vi "Target.vi"() -> ()   [LabVIEW 2025]
uses:
  <vilib>/Platform/TimedLoop/XDataNode/timing_clust.ctl
  <vilib>/Platform/TimedLoop/XDataNode/nitl_modes.ctl
  <vilib>/Platform/TimedLoop/XDataNode/wakeup.ctl
  <vilib>/rvi/Emulation/niFpgaSctlEmulationGetInTimedLoop.vi
  <vilib>/rvi/Emulation/niFpgaEmulationReportErrorSimple.vi
  <vilib>/rvi/Emulation/niFpgaGetClockAttributes.vi
  <vilib>/rvi/Emulation/niFpgaCriticalErrorInLSC.vi
  <vilib>/rvi/linearAlgebra/MatrixMultiply/simVIs/SubVI/nifxpla_MatrixMultiply_SimMatrixSizes.vi
  <vilib>/rvi/linearAlgebra/MatrixMultiply/simVIs/SubVI/nifxpla_MatrixMultiply_Sim4WireAdapterVector.vi
  <vilib>/rvi/linearAlgebra/MatrixMultiply/simVIs/SubVI/nifxpla_MatrixMultiply_SimFrameHandShake.vi
  <vilib>/rvi/linearAlgebra/MatrixMultiply/simVIs/SubVI/nifxpla_MatrixMultiply_SimEndlessCounter.vi
  <vilib>/rvi/linearAlgebra/MatrixMultiply/simVIs/SubVI/nifxpla_MatrixMultiply_SimVectorDataBuffer.vi
  <vilib>/rvi/ClientSDK/Core/DevComputerLib/Private/Multiply(dfxp64).vi
  <vilib>/rvi/ClientSDK/Core/DevComputerLib/Private/Dfxp128ToDfxp256.vi
  <vilib>/rvi/ClientSDK/Core/DevComputerLib/Private/Add(dfxp256).vi
  <vilib>/rvi/ClientSDK/Core/DevComputerLib/Private/Subtract(dfxp256).vi
  <vilib>/rvi/ClientSDK/Core/DevComputerLib/Private/ToDfxp64(dfxp256).vi
  <vilib>/platform/TimedLoop/XDataNode/XDataNode.xnode
  <vilib>/rvi/linearAlgebra/MatrixMultiply/XNode/nifxpla_MatrixMultiply.xnode
  <vilib>/rvi/linearAlgebra/MatrixMultiply/simVIs/nifxpla_MatrixMultiply_SimTemplateEinEout.vi
  <vilib>/rvi/linearAlgebra/MatrixMultiply/simVIs/nifxpla_MatrixMultiply_SimTemplateEinVout.vi
  <vilib>/rvi/linearAlgebra/MatrixMultiply/simVIs/nifxpla_MatrixMultiply_SimTemplateVinEout.vi
  <vilib>/rvi/linearAlgebra/MatrixMultiply/simVIs/nifxpla_MatrixMultiply_SimTemplateVinVout.vi
  <vilib>/Platform/TimedLoop/XDataNode/XDNodeRunTimeDep.lvlib
panel:
  out "C1+B":fxp<+/-,33,17>[](array[numeric])
  out "C1":fxp<+/-,32,16>[](array[numeric])
  out "Cycle Count":i32
  out "C2+B":fxp<+/-,33,17>[](array[numeric])
  out "C2":fxp<+/-,32,16>[](array[numeric])
  out "Cycle Count 2":i32
  out "C3+B":fxp<+/-,33,17>[](array[numeric])
  out "C3":fxp<+/-,32,16>[](array[numeric])
  out "Cycle Count 3":i32
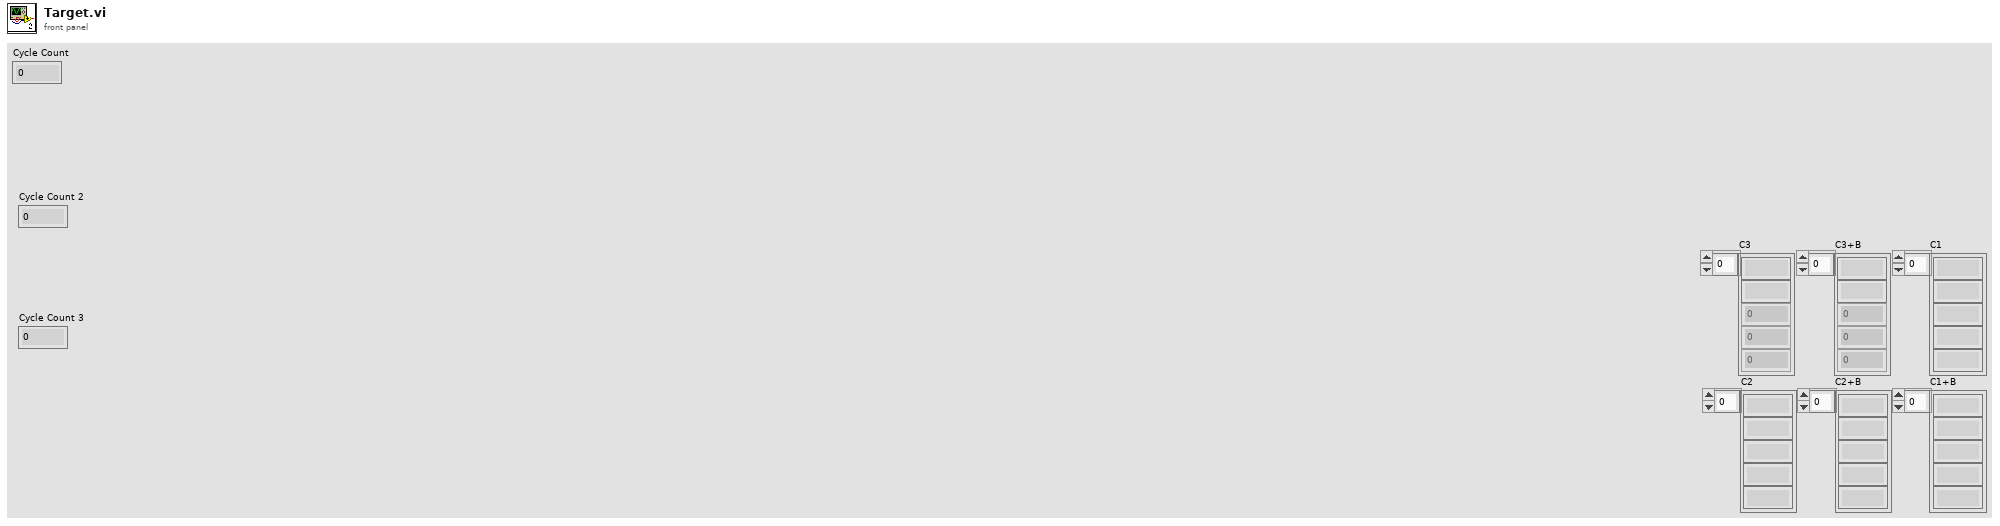
[diagram p1: front panel]
types:
  T1 = typedef "XDNodeRunTimeDep.lvlib/timing_clust.ctl" = cluster{"Expected End [f-1]":u64, "Actual End [f-1]":u64, "Finished Late? [f-1]":bool, "Expected End [i-1]":u64, "Actual End [i-1]":u64, "Finished Late? [i-1]":bool, "Expected Start [i]":u64, "Actual Start [i]":u64, "Expected Start [f]":u64, "Actual Start [f]":u64, "Source Name":string, "Structure Name":string, "Period":i64, "Deadline":i64, "Offset":i64, "Start":i64, "Priority":i32, "Timeout":i32, "Mode":T2, "Wakeup Reason":T3, "Error":errorcluster, "Source Type":string, "Secondary Source Type":string, "Global End Time":u64, "Global Start Time":u64, "Frame Duration":u64, "Iteration Duration":u64, "Assigned CPU":i32, "I/O Scan Engine Mode":u32}
  T2 = typedef "XDNodeRunTimeDep.lvlib/nitl_modes.ctl" = enum32{"No Change", "Process missed periods, maintain original phase", "Discard missed periods, maintain original phase", "Process missed periods, ignore original phase", "Discard missed periods, ignore original phase"}
  T3 = typedef "XDNodeRunTimeDep.lvlib/wakeup.ctl" = enum32{"Normal", "Aborted", "Asynchronous wakeup", "Timing source error", "Timed loop error", "Timeout"}
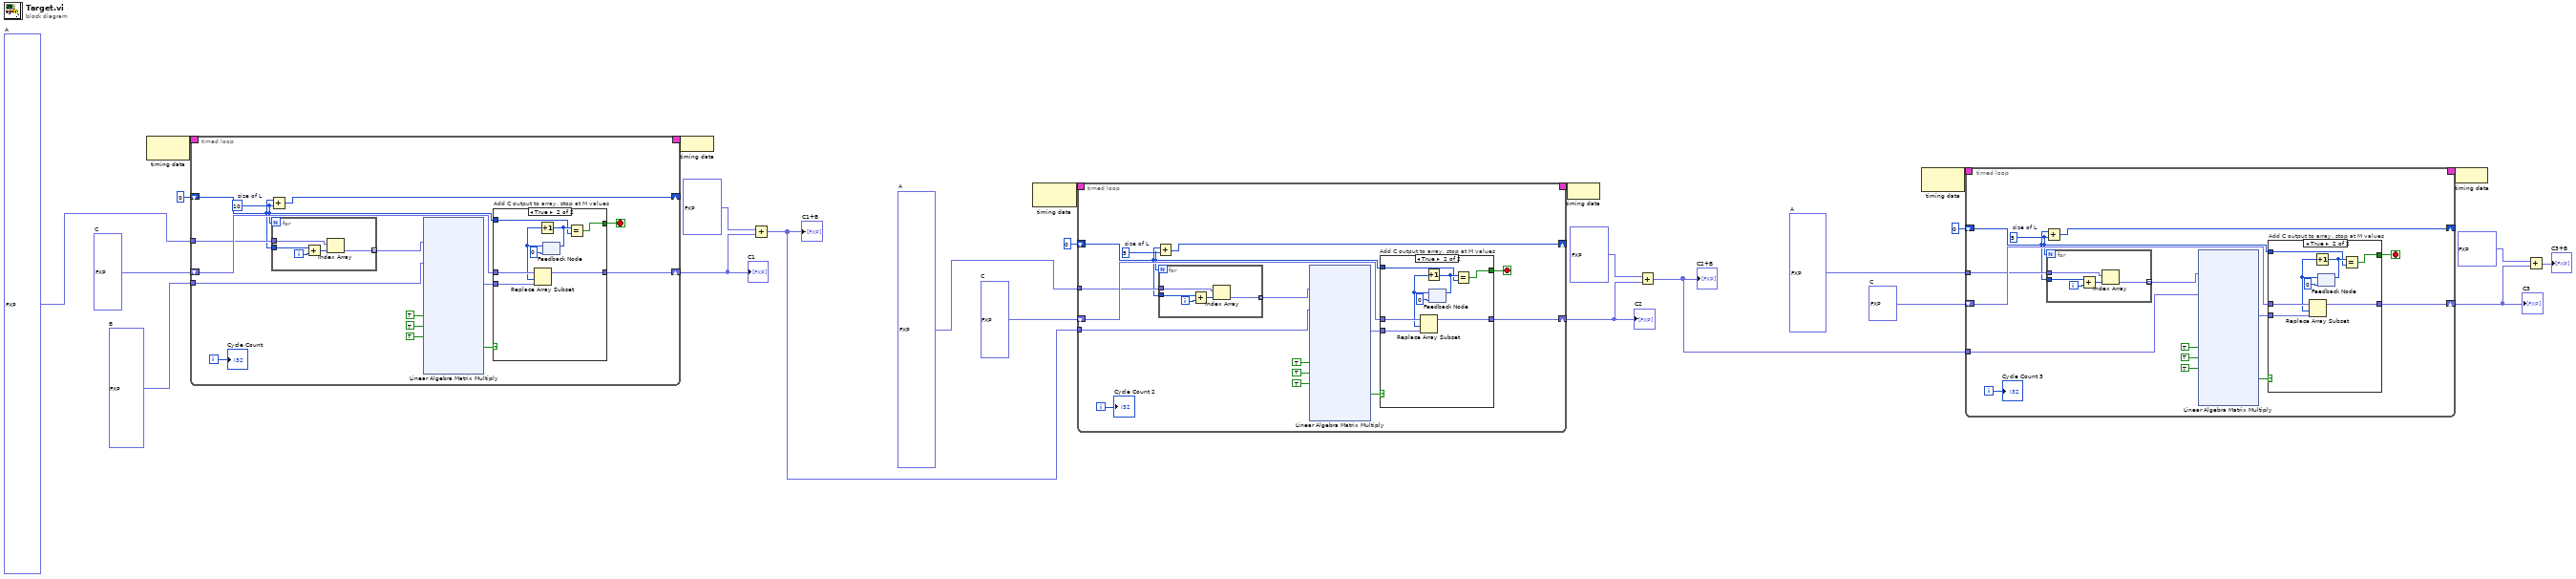
[diagram p0: block diagram]
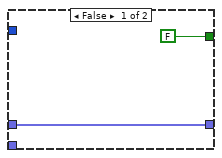
[diagram p2: hidden frame]
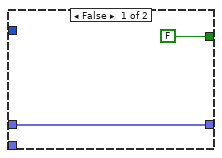
[diagram p3: hidden frame]
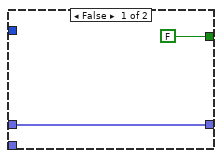
[diagram p4: hidden frame]
diagram:
  w17 = fxp<+/-,32,16>[] [1.0, 2.0, 3.0, 4.0, 5.0, 6.0, 7.0, 8.0, 9.0, 10.0, 11.0, 12.0, 13.0, 14.0, 15.0, 16.0, 17.0, 18.0, 19.0, 20.0, 21.0, 22.0, 23.0, 24.0, 25.0, 26.0, 27.0, 28.0, 29.0, 30.0, 31.0, 32.0, 33.0, 34.0, 35.0, 36.0, 37.0, 38.0, 39.0, 40.0, 41.0, 42.0, 43.0, 44.0, 45.0, 46.0, 47.0, 48.0, 49.0, 50.0]  # A
  w18 = fxp<+/-,32,16>[] [1.0, 2.0, 3.0, 4.0, 5.0, 6.0, 7.0, 8.0, 9.0, 10.0]  # B
  w19 = fxp<+/-,32,16>[] [0.0, 0.0, 0.0, 0.0, 0.0]  # C
  w12 = fxp<+/-,32,16>[] [1.0, 2.0, 3.0, 4.0, 5.0, 6.0, 7.0, 8.0, 9.0, 10.0, 11.0, 12.0, 13.0, 14.0, 15.0, 16.0, 17.0, 18.0, 19.0, 20.0, 21.0, 22.0, 23.0, 24.0, 25.0]  # A
  w13 = fxp<+/-,32,16>[] [0.0, 0.0, 0.0, 0.0, 0.0]  # C
  w7 = fxp<+/-,32,16>[] [1.0, 2.0, 3.0, 4.0, 5.0, 6.0, 7.0, 8.0, 9.0, 10.0]  # A
  w8 = fxp<+/-,32,16>[] [0.0, 0.0]  # C
  n1 = node-c288() -> (w21:T1)  [unwired: 1 in]
  n2 = timed-loop {
    timing: w21 -> [_]
    timing-out: [_] -> w20
    shift-right: [w39] -> w15
    shift-left: w19 -> [w38]
    tunnel: w18 -> [w33]
    tunnel: w17 -> [w36]
    shift-right: [w27] -> _
    shift-left: 0 ("length") -> [w29]
    i -> [w34]
    stop <- w37 stop-if-true
    w28 = 10  # size of L
    n3 = Add(x=w29, y=w28) -> (x+y=w27:i32)
    n4 = for {
      N: w28 -> [_]
      tunnel: w36 -> [w45]
      tunnel: w29 -> [w43]
      tunnel: [w41] -> w31 mode=indexing
      i -> [w44]
      n5 = Add(x=w43, y=w44) -> (x+y=w42:i32)
      n6 = Index Array "Index Array"(array=w45, index=w42) -> (element=w41:fxp<+/-,32,16>)
    }
    n7 = xnode ("Linear Algebra Matrix Multiply")("ar"=w31, "br"=w33, "a valid"=TRUE, "b valid"=TRUE, "ready for output (T)"=TRUE) -> ("cr"=w32:fxp<+/-,32,16>[], "output valid"=w26:bool)  [unwired: 2 in, 4 out]
    n8 = case "Add C output to array, stop at M values" shown="True" w26 {
      tunnel: w32 -> [_ w51]
      tunnel: [w47 w54] -> w39
      tunnel: w38 -> [w47 w55]
      tunnel: [FALSE w52] -> w37
      tunnel: w28 -> [_ w48]
      frame False {
      }
      frame True {
        n9 = feedback #1(0 ("x")) -> (w50:i32)
        n10 = Replace Array Subset(array=w55, new element=w51, index=w50) -> (w54:fxp<+/-,32,16>[])
        n11 = Increment(x=w50) -> (x+1=w49:i32)
        n12 = feedback-in #1(w49) -> ()
        n13 = Equal?(x=w49, y=w48) -> (x = y?=w52:bool)
      }
    }
    "Cycle Count" <- w34
  }
  "C1" <- w15
  n14 = node-c288(w20) -> ()
  n15 = Add(x=fxp<+/-,32,16>[] [0.5, 0.5, 0.5, 0.5, 0.5], y=w15) -> (x+y=w2:fxp<+/-,33,17>[])
  "C1+B" <- w2
  n16 = node-c288() -> (w23:T1)  [unwired: 1 in]
  n17 = timed-loop {
    timing: w23 -> [_]
    timing-out: [_] -> w22
    shift-right: [w71] -> w10
    shift-left: w13 -> [w70]
    tunnel: w2 -> [w65]
    tunnel: w12 -> [w68]
    shift-right: [w59] -> _
    shift-left: 0 ("length") -> [w61]
    i -> [w66]
    stop <- w69 stop-if-true
    w60 = 5  # size of L
    n18 = Add(x=w61, y=w60) -> (x+y=w59:i32)
    n19 = for {
      N: w60 -> [_]
      tunnel: w68 -> [w77]
      tunnel: w61 -> [w75]
      tunnel: [w73] -> w63 mode=indexing
      i -> [w76]
      n20 = Add(x=w75, y=w76) -> (x+y=w74:i32)
      n21 = Index Array "Index Array"(array=w77, index=w74) -> (element=w73:fxp<+/-,32,16>)
    }
    n22 = xnode ("Linear Algebra Matrix Multiply")("ar"=w63, "br"=w65, "a valid"=TRUE, "b valid"=TRUE, "ready for output (T)"=TRUE) -> ("cr"=w64:fxp<+/-,32,16>[], "output valid"=w58:bool)  [unwired: 2 in, 4 out]
    n23 = case "Add C output to array, stop at M values" shown="True" w58 {
      tunnel: w64 -> [_ w83]
      tunnel: [w79 w86] -> w71
      tunnel: w70 -> [w79 w87]
      tunnel: [FALSE w84] -> w69
      tunnel: w60 -> [_ w80]
      frame False {
      }
      frame True {
        n24 = feedback #2(0 ("x")) -> (w82:i32)
        n25 = Replace Array Subset(array=w87, new element=w83, index=w82) -> (w86:fxp<+/-,32,16>[])
        n26 = Increment(x=w82) -> (x+1=w81:i32)
        n27 = feedback-in #2(w81) -> ()
        n28 = Equal?(x=w81, y=w80) -> (x = y?=w84:bool)
      }
    }
    "Cycle Count 2" <- w66
  }
  "C2" <- w10
  n29 = node-c288(w22) -> ()
  n30 = Add(x=fxp<+/-,32,16>[] [0.5, 0.5, 0.5, 0.5, 0.5], y=w10) -> (x+y=w1:fxp<+/-,33,17>[])
  "C2+B" <- w1
  n31 = node-c288() -> (w25:T1)  [unwired: 1 in]
  n32 = timed-loop {
    timing: w25 -> [_]
    timing-out: [_] -> w24
    shift-right: [w103] -> w5
    shift-left: w8 -> [w102]
    tunnel: w7 -> [w100]
    shift-right: [w92] -> _
    shift-left: 0 ("length") -> [w94]
    tunnel: w1 -> [w90]
    i -> [w98]
    stop <- w101 stop-if-true
    w93 = 5  # size of L
    n33 = Add(x=w94, y=w93) -> (x+y=w92:i32)
    n34 = for {
      N: w93 -> [_]
      tunnel: w100 -> [w109]
      tunnel: w94 -> [w107]
      tunnel: [w105] -> w96 mode=indexing
      i -> [w108]
      n35 = Add(x=w107, y=w108) -> (x+y=w106:i32)
      n36 = Index Array "Index Array"(array=w109, index=w106) -> (element=w105:fxp<+/-,32,16>)
    }
    n37 = xnode ("Linear Algebra Matrix Multiply")("ar"=w96, "br"=w90, "a valid"=TRUE, "b valid"=TRUE, "ready for output (T)"=TRUE) -> ("cr"=w97:fxp<+/-,32,16>[], "output valid"=w91:bool)  [unwired: 2 in, 4 out]
    n38 = case "Add C output to array, stop at M values" shown="True" w91 {
      tunnel: w97 -> [_ w115]
      tunnel: [w111 w118] -> w103
      tunnel: w102 -> [w111 w119]
      tunnel: [FALSE w116] -> w101
      tunnel: w93 -> [_ w112]
      frame False {
      }
      frame True {
        n39 = feedback #3(0 ("x")) -> (w114:i32)
        n40 = Replace Array Subset(array=w119, new element=w115, index=w114) -> (w118:fxp<+/-,32,16>[])
        n41 = Increment(x=w114) -> (x+1=w113:i32)
        n42 = feedback-in #3(w113) -> ()
        n43 = Equal?(x=w113, y=w112) -> (x = y?=w116:bool)
      }
    }
    "Cycle Count 3" <- w98
  }
  "C3" <- w5
  n44 = node-c288(w24) -> ()
  n45 = Add(x=fxp<+/-,32,16>[] [0.5, 0.5], y=w5) -> (x+y=→"C3+B":fxp<+/-,33,17>[])
